vi "Initialize Andor.vi"() -> (0 "Error Out 2":errorcluster, 1 "Drv Success?":i32)   [LabVIEW 2014]
uses:
  Initilize Globals.vi
  lib/Andorlib/atmcd32d.lvlib
panel:
  out "String":string
  out "HS Speed":dbl format="%#_13g"
  out "Number HS Speeds":i32
  out "VS Speed":dbl format="%#_13g"
  out "Number VS Speeds":i32
  out "Camera FirmWare Version":i32
  out "Y-pixels":u32
  out "X-pixels":u32
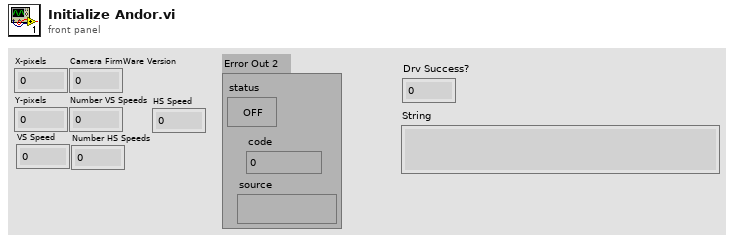
[diagram p1: front panel]
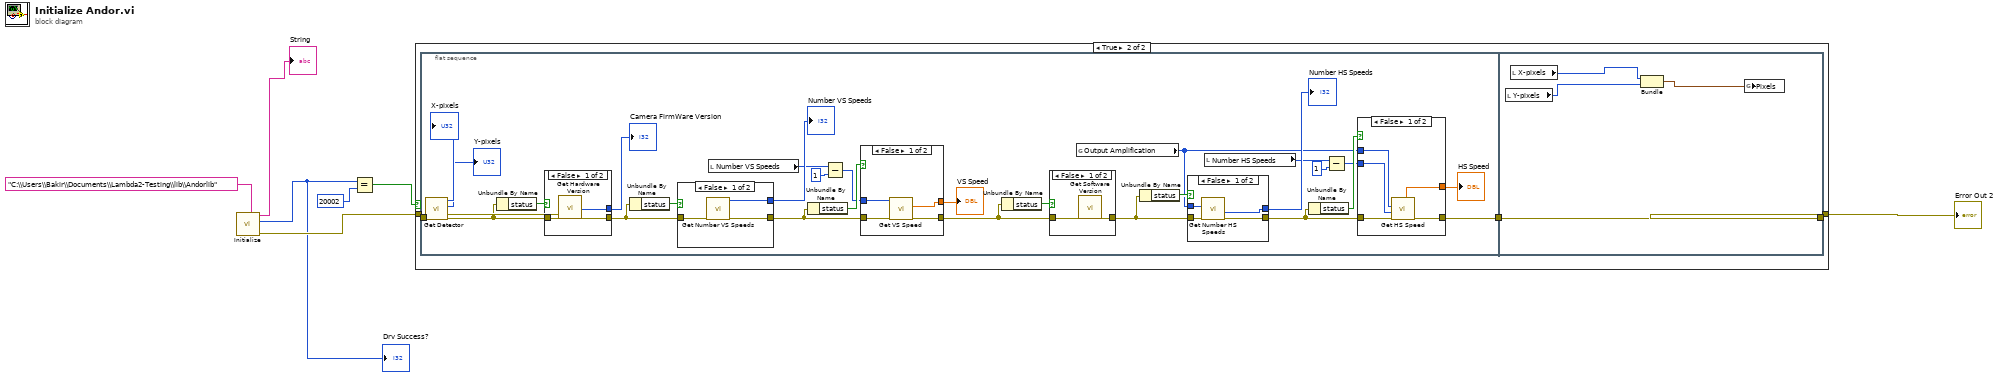
[diagram p0: block diagram]
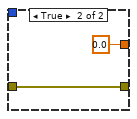
[diagram p3: hidden frame]
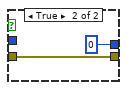
[diagram p4: hidden frame]
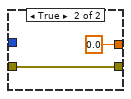
[diagram p6: hidden frame]
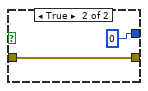
[diagram p7: hidden frame]
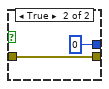
[diagram p8: hidden frame]
diagram:
  n1 = call "Initialize.vi"("dir"="C:\\Users\\Bakir\\Documents\\Lambda2-Testing\\lib\\Andorlib") -> ("error out"=w6:errorcluster, "function return"=w1:u32, "dir out"=→"String":string)  [unwired: 8 in]
  "Drv Success?" <- w1
  n2 = Equal?(x=w1, y=20002) -> (x = y?=w2:bool)
  n3 = case shown="True" w2 {
    tunnel: [w8 w10] -> w7
    tunnel: w6 -> [w8 w11]
    frame False {
    }
    frame True {
      n4 = flat-sequence {
        tunnel: w11 -> [w39]
        tunnel: [w27] -> w9
        tunnel: [w75] -> w10
        tunnel: w9 -> [w75]
        frame #0 {
          n5 = call "Get Detector.vi"("error in (no error)"=w39) -> ("error out"=w32:errorcluster, "ypixels out"=→"Y-pixels":i32, "xpixels out"=→"X-pixels":i32)  [unwired: 7 in, 1 out]
          n6 = Unbundle By Name(w32) -> ("status"=w38:bool)
          n7 = case shown="False" w38 {
            tunnel: w32 -> [w69 w71]
            tunnel: [w68 w71] -> w31
            tunnel: [w67 0] -> w23
            frame False {
              n8 = call "Get Hardware Version.vi"("error in (no error)"=w69) -> ("CameraFirmwareVersion out"=w67:u32, "error out"=w68:errorcluster)  [unwired: 19 in, 6 out]
            }
            frame True {
            }
          }
          "Camera FirmWare Version" <- w23
          n9 = Unbundle By Name(w31) -> ("status"=w37:bool)
          n10 = case shown="False" w37 {
            tunnel: w31 -> [w64 w66]
            tunnel: [w63 w66] -> w30
            tunnel: [w62 0] -> w22
            frame False {
              n11 = call "Get Number VS Speeds.vi"("error in (no error)"=w64) -> ("error out"=w63:errorcluster, "speeds out"=w62:i32)  [unwired: 8 in, 1 out]
            }
            frame True {
            }
          }
          "Number VS Speeds" <- w22
          n12 = local read "Number VS Speeds"() -> (w21:i32)
          n13 = Unbundle By Name(w30) -> ("status"=w36:bool)
          n14 = Subtract(x=w21, y=1) -> (x-y=w19:i32)
          n15 = case shown="False" w36 {
            tunnel: w30 -> [w58 w61]
            tunnel: [w59 w61] -> w29
            tunnel: w19 -> [w57 _]
            tunnel: [w56 0.0] -> w18
            frame False {
              n16 = call "Get VS Speed.vi"("error in (no error)"=w58, "index"=w57) -> ("error out"=w59:errorcluster, "speed out"=w56:sgl)  [unwired: 7 in, 1 out]
            }
            frame True {
            }
          }
          "VS Speed" <- w18
          n17 = Unbundle By Name(w29) -> ("status"=w35:bool)
          n18 = case shown="False" w35 {
            tunnel: w29 -> [w54 w55]
            tunnel: [w53 w55] -> w28
            frame False {
              n19 = call "Get Software Version.vi"("error in (no error)"=w54) -> ("error out"=w53:errorcluster)  [unwired: 19 in, 7 out]
            }
            frame True {
            }
          }
          n20 = global read "Initilize Globals.vi" "Output Amplification"() -> (w16:i32)
          n21 = Unbundle By Name(w28) -> ("status"=w34:bool)
          n22 = case shown="False" w34 {
            tunnel: w28 -> [w50 w52]
            tunnel: [w49 w52] -> w26
            tunnel: w16 -> [w48 _]
            tunnel: [w47 0] -> w17
            frame False {
              n23 = call "Get Number HS Speeds.vi"("error in (no error)"=w50, "typ"=w48) -> ("error out"=w49:errorcluster, "speeds out"=w47:i32)  [unwired: 7 in, 1 out]
            }
            frame True {
            }
          }
          "Number HS Speeds" <- w17
          n24 = local read "Number HS Speeds"() -> (w15:i32)
          n25 = Unbundle By Name(w26) -> ("status"=w33:bool)
          n26 = Subtract(x=w15, y=1) -> (x-y=w13:i32)
          n27 = case shown="False" w33 {
            tunnel: w26 -> [w44 w46]
            tunnel: [w43 w46] -> w27
            tunnel: w16 -> [w42 _]
            tunnel: w13 -> [w41 _]
            tunnel: [w40 0.0] -> w12
            frame False {
              n28 = call "Get HS Speed.vi"("error in (no error)"=w44, "index"=w41, "typ"=w42) -> ("error out"=w43:errorcluster, "speed out"=w40:sgl)  [unwired: 6 in, 1 out]
            }
            frame True {
            }
          }
          "HS Speed" <- w12
        }
        frame #1 {
          n29 = local read "Y-pixels"() -> (w72:u32)
          n30 = local read "X-pixels"() -> (w73:u32)
          n31 = Bundle("X-pixels"=w73, "Y-pixels"=w72) -> (w74:cluster{"X-pixels":u32, "Y-pixels":u32})  [unwired: 1 in]
          n32 = global write "Initilize Globals.vi" "Pixels"(w74) -> ()
        }
      }
    }
  }
  "Error Out 2" <- w7
